vi "Demo 1 - Image Gallery - Get Mouse X Axis Position.vi"(8 "Error In":errorcluster) -> (0 "Error Out":errorcluster, 3 "Mouse X Axis Out":i32)   [LabVIEW 2011]
uses:
  <vilib>/Utility/inputDevices.llb/mouseAcquire.vi
  <vilib>/Utility/inputDevices.llb/closeMouse.vi
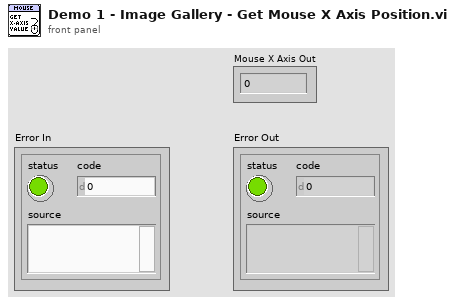
[diagram p1: front panel]
types:
  T1 = cluster{"Horizontal":i32, "Vertical":i32, "Scrolling":i32}
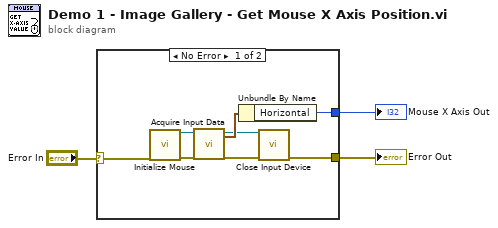
[diagram p0: block diagram]
diagram:
  n1 = case shown="No Error" "Error In" {
    selector: "Error In" -> [w4 w12]
    tunnel: [w8 _] -> w3
    tunnel: [w6 w12] -> w2
    frame No Error {
      n2 = call <vilib>:"Initialize Mouse.vi"("error in (no error)"=w4) -> ("error out"=w9:errorcluster, "device ID"=w10:refnum<k1>)  [unwired: 9 in]
      n3 = call-poly <vilib>:"Acquire Input Data.vi"("device ID"=w10, "error in (no error)"=w9) -> ("device ID"=w5:refnum<k1>, "axis info"=w11:T1, "error out"=w7:errorcluster)  [unwired: 14 in, 1 out]
      n4 = Unbundle By Name(w11) -> ("Horizontal"=w8:i32)
      n5 = call-poly <vilib>:"Close Input Device.vi"("error in (no error)"=w7, "device ID"=w5) -> ("error out"=w6:errorcluster)  [unwired: 8 in]
    }
    frame Error {
    }
  }
  "Mouse X Axis Out" <- w3
  "Error Out" <- w2
